vi "DAQNavi Is Task Done.vi"(3 "error in (no error)":errorcluster, 5 "task in":i32) -> (0 "error out":errorcluster, 1 "isTaskDone":bool, 2 "task out":i32)   [LabVIEW 2020]
doc: "You can use the Is Task Done function/VI for applications in which you need to monitor the progress of a task running in one section of your application from another section of your application.\nIn general, use the Is Task Done function/VI with continuous measurements and generations when you are not actively reading or writing samples but want to monitor for errors."
uses:
  DAQNavi_LV.dll
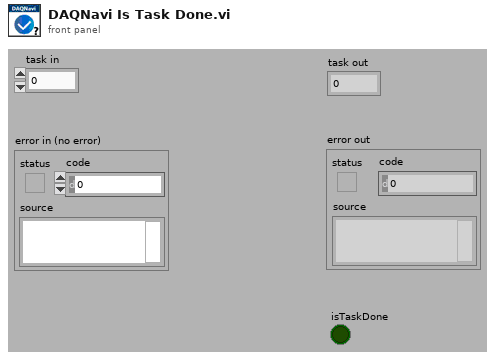
[diagram p1: front panel]
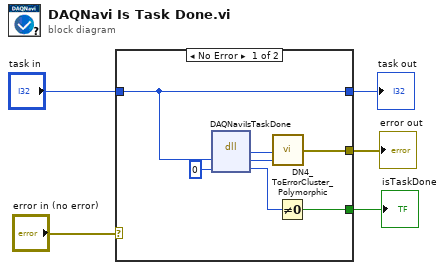
[diagram p0: block diagram]
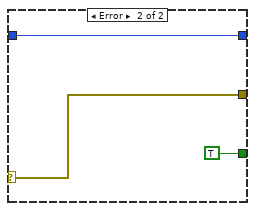
[diagram p2: hidden frame]
diagram:
  n1 = case shown="No Error" "error in (no error)" {
    selector: "error in (no error)" -> [_ w15]
    tunnel: "task in" -> [w9 w14]
    tunnel: [w10 TRUE] -> w3
    tunnel: [w9 w14] -> w2
    tunnel: [w8 w15] -> w1
    frame No Error {
      n2 = dll-call lib="DAQNavi_LV.dll" fn="DAQNaviIsTaskDone"("taskID"=w9, "isTaskDone"=i8 0) -> ("return type"=w7:i32, "taskID"=w6:i32, "isTaskDone"=w11:i8)  [unwired: 3 in, 2 out]
      n3 = call "DN4_ToErrorCluster_Polymorphic.vi"("task id"=w6, "error code"=w7) -> ("error out"=w8:errorcluster)  [unwired: 3 out]
      n4 = Not Equal To 0?(x=w11) -> (x != 0?=w10:bool)
    }
    frame Error {
    }
  }
  "task out" <- w2
  "error out" <- w1
  "isTaskDone" <- w3
